vi "Signal Math (V1.00).vi"(0 "Time Data":refnum<class "GSwFormDSP.lvclass">, 5 "error in (no error)":errorcluster, 7 "Application Name":string="SigMath", 9 "State Queue":T2[](array[typedef])=["SC >>> Initialize"]) -> (19 "error out":errorcluster)   [LabVIEW 2022 SP3, in "SigMath.lvclass"]
uses:
  SigMath.lvclass
  API/Generic Utilities_class/utils/GenUtil State List.ctl
  API/GSwFormDSP_class/GSwFormDSP.lvclass
  <vilib>/Utility/sysdir.llb/System Directory Type.ctl
  W:/projects/archives/23 Charette AI Group/SPWB/API/Generic Utilities_class/Generic Utilities.lvclass
  <vilib>/Platform/browser.llb/Open URL in Default Browser (path).vi
  <vilib>/addons/_AddQ/G#Object/G#Object.lvclass
  API/Generic Utilities_class/Generic Utilities.lvclass
panel:
  in  "Operation":T1(tab)
  in  "Add Signals":bool
  in  "Add - Select Signals":i32[](listbox) caption="Select Signals"
  in  "Deconvolute Signals":bool
  in  "Convolute Signals":bool
  in  "Substract Signals":bool
  in  "Sub Signals A":i32[](listbox) caption="Select Signals (Set A)"
  in  "Sub Signals B":i32[](listbox) caption="Select Signals (Set B)"
  out "Measured Delay (Samples)":dbl
  out "Measured Delay (msec)":dbl
  in  "Weighting":u16(ring) items=["biased (N)", "unbiased (N-k)"]
  out "Cross Correlation Graph":cluster{"Ramp Pattern":dbl[], "Rxy":dbl[]}(graph)
  in  "X-Corr Signals A":i32[](listbox) caption="Select Signals (Set A)"
  in  "X-Corr Signals B":i32[](listbox) caption="Select Signals (Set B)"
  in  "AppData Folder":bool
  out "State History":string[](array[string])
  out "State Index":i32
  in  "Exit":bool
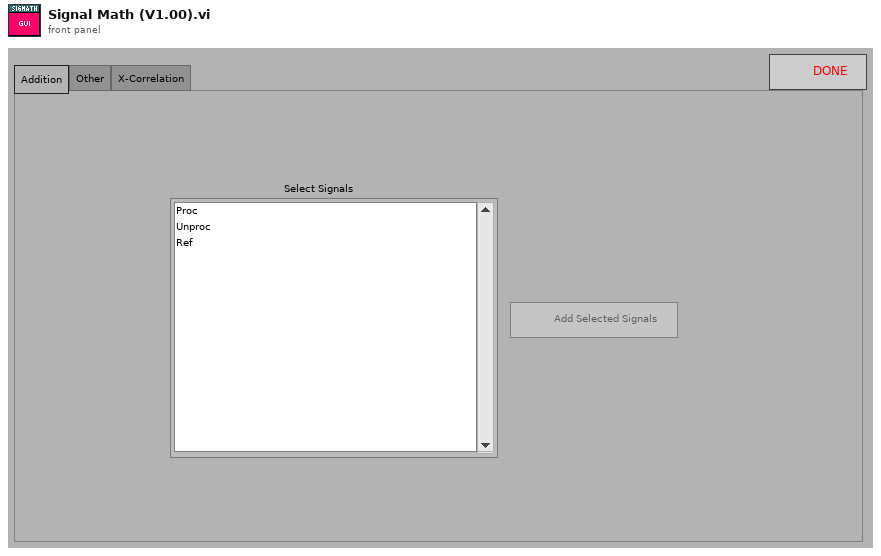
[diagram p1: front panel]
types:
  T1 = enum32{"Addition", "Other", "X-Correlation", "Settings"}
  T2 = typedef "Generic Utilities.lvclass/GenUtil State List.ctl" = string
  T3 = enum8{"Enabled", "Disabled", "Disabled and Grayed Out"}
  T4 = enum32{"Invalid", "Standard", "Closed", "Hidden", "Minimized", "Maximized"}
  T5 = typedef "System Directory Type.ctl" = i32
  T6 = typedef "SigMath.lvclass/SigMath Data.ctl" = cluster{"New Time Data Obj?":bool, "GSwFormDSP":refnum<class "GSwFormDSP.lvclass">}
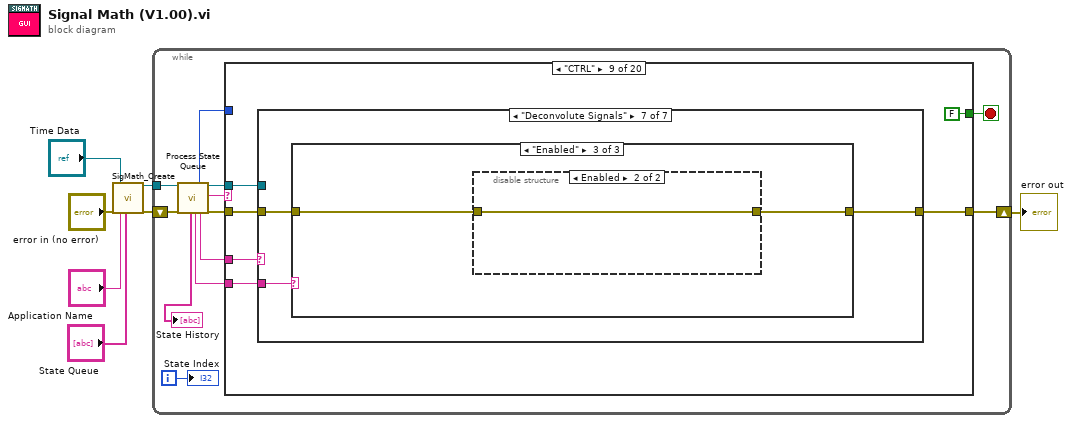
[diagram p0: block diagram]
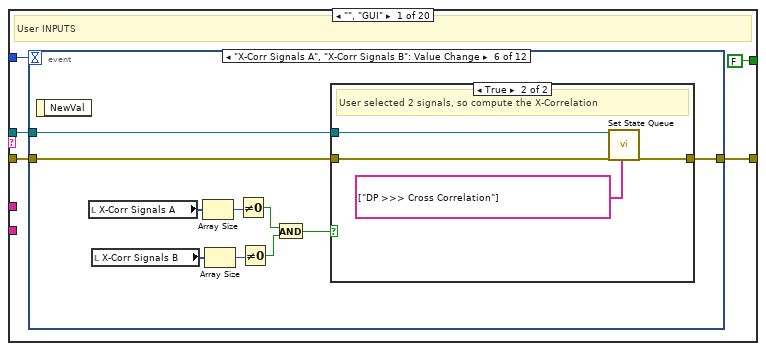
[diagram p2: hidden frame]
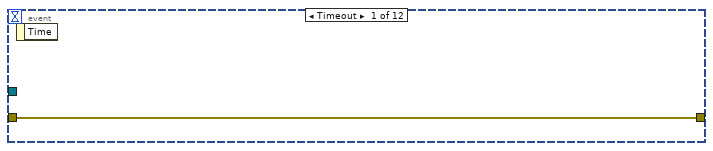
[diagram p3: hidden frame]
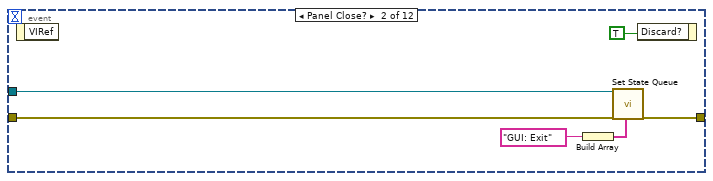
[diagram p4: hidden frame]
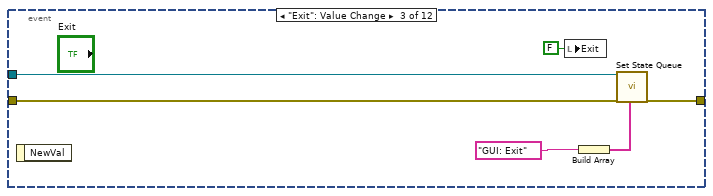
[diagram p5: hidden frame]
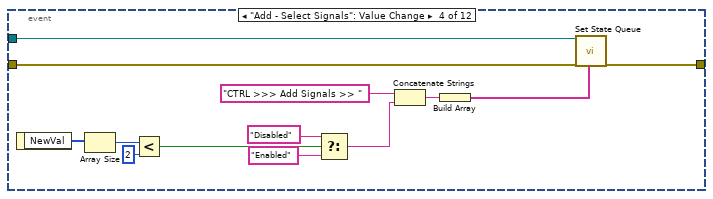
[diagram p6: hidden frame]
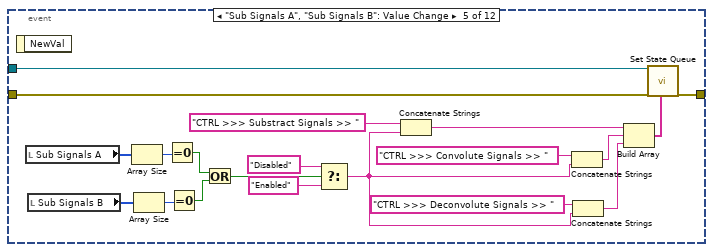
[diagram p7: hidden frame]
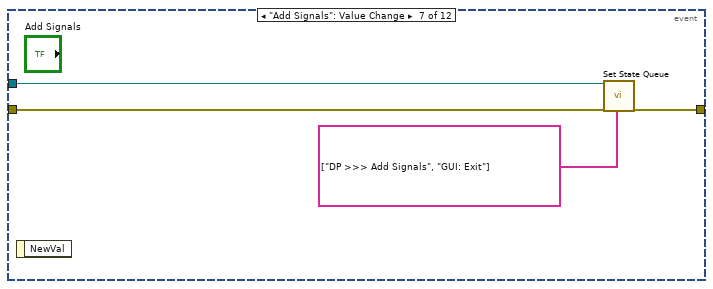
[diagram p9: hidden frame]
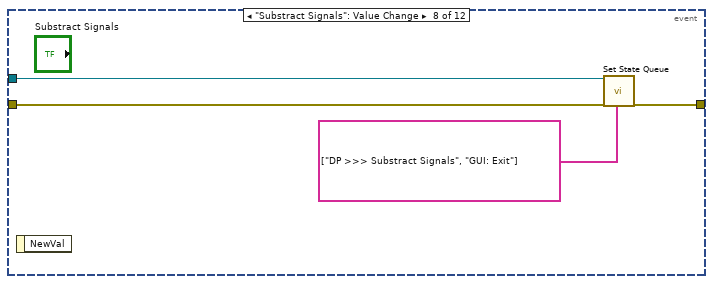
[diagram p10: hidden frame]
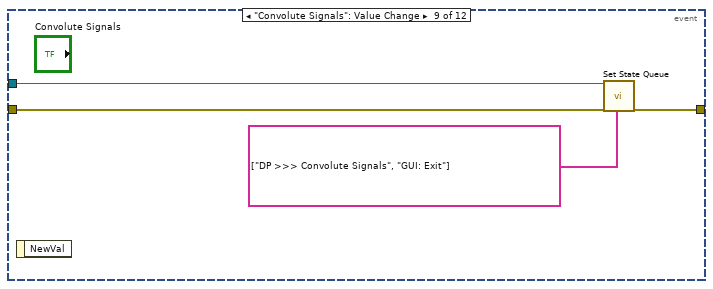
[diagram p11: hidden frame]
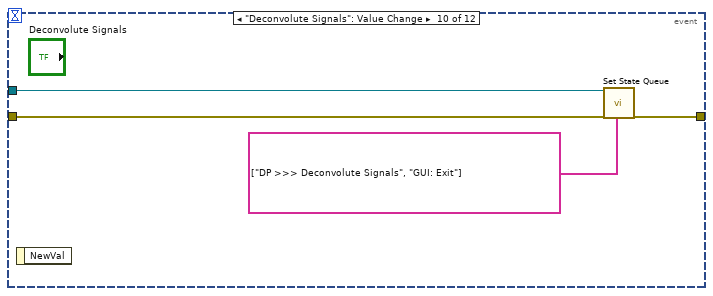
[diagram p12: hidden frame]
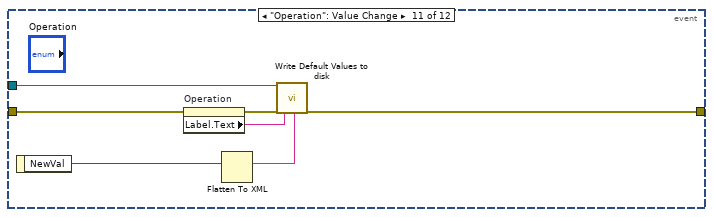
[diagram p13: hidden frame]
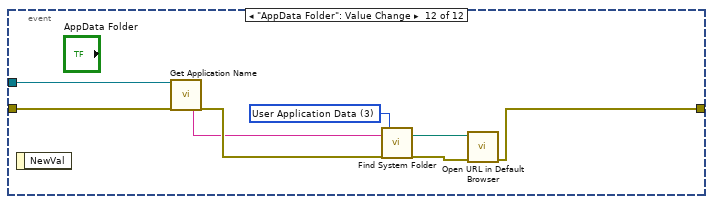
[diagram p14: hidden frame]
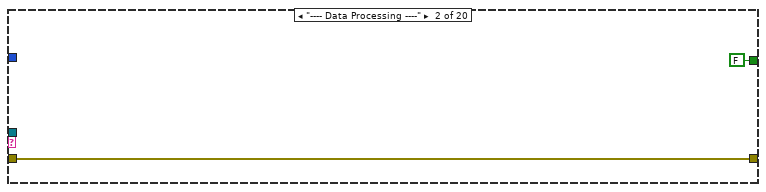
[diagram p15: hidden frame]
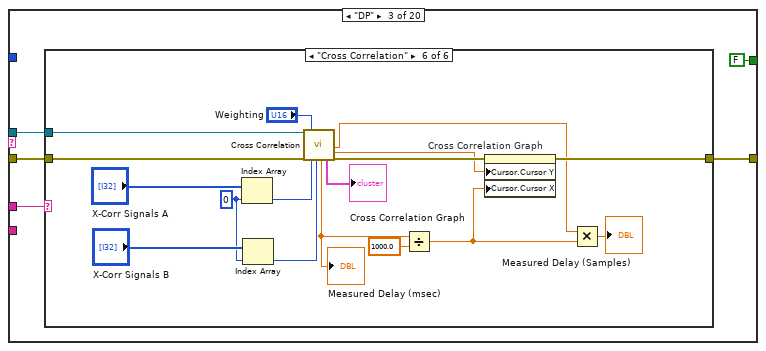
[diagram p16: hidden frame]
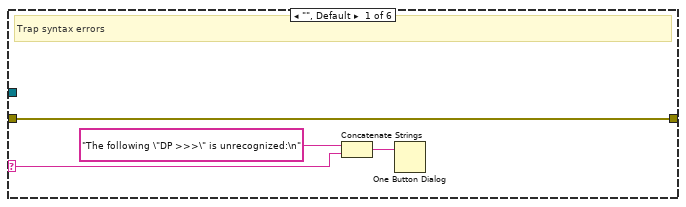
[diagram p17: hidden frame]
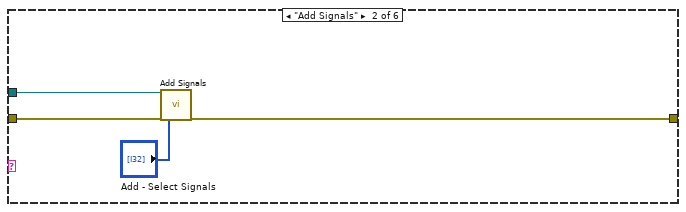
[diagram p18: hidden frame]
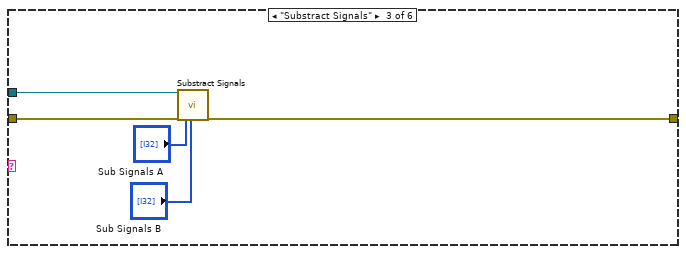
[diagram p19: hidden frame]
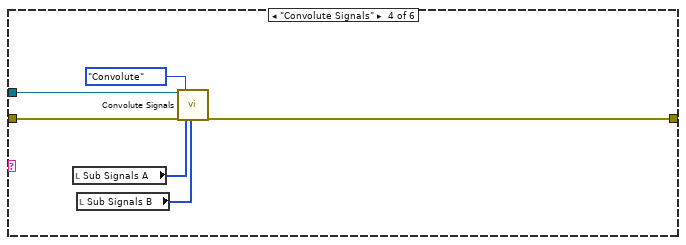
[diagram p20: hidden frame]
diagram:
  n1 = call "SigMath_Create.vi"("error in (no error)"="error in (no error)", "Time Data"="Time Data", "Application Name"="Application Name", "State Queue"="State Queue") -> ("reference out"=w7:refnum<class "SigMath.lvclass">, "error out"=w6:errorcluster)  [unwired: 14 in]
  n2 = while {
    shift-right: [w11] -> w2
    shift-left: w6 -> [w16]
    tunnel: w7 -> [w17]
    i -> [w18]
    stop <- w19 stop-if-true
    n3 = call "Process State Queue.vi"("reference in"=w17, "error in (no error)"=w16) -> ("State History"=→"State History":string[], "Additional Options"=w8:string, "Timeout"=w15:i32, "State Option"=w10:string, "reference out"=w14:refnum<class "SigMath.lvclass">, "Current State"=w13:string, "error out"=w12:errorcluster)  [unwired: 10 in, 1 out]
    n4 = case shown="\"CTRL\"" w13 {
      selector: w13 -> [_ _ _ _ _ _ _ _ _ _ _ _ _ _ _ _ w449 _ _ _]
      tunnel: w14 -> [w22 _ w119 _ w168 _ w184 _ w196 w317 _ w353 w372 w408 w433 _ _ _ _ w459]
      tunnel: [FALSE FALSE FALSE FALSE FALSE FALSE FALSE FALSE FALSE FALSE FALSE FALSE TRUE FALSE FALSE FALSE FALSE FALSE FALSE TRUE] -> w19
      tunnel: w15 -> [w23 _ _ _ _ _ _ _ _ _ _ _ _ _ _ _ _ _ _ _]
      tunnel: w10 -> [_ _ w122 _ w171 _ w180 _ w197 w314 _ _ _ w417 _ _ _ _ _ _]
      tunnel: w12 -> [w21 w117 w121 w166 w169 w177 w183 w191 w194 w316 w337 w350 w369 w407 w434 w445 w447 w452 w455 w458]
      tunnel: [w20 w117 w120 w166 w170 w177 w182 w191 w195 w315 w337 w342 w368 w405 w430 w445 w447 errorcluster {"status"=FALSE, "code"=0, "source"=""} ("error out") w455 w457] -> w11
      tunnel: w8 -> [_ _ _ _ _ _ _ _ w193 _ _ _ _ _ _ _ _ _ _ _]
      frame "", "GUI" {
        # "User INPUTS"
        n5 = event shown="[5] \"X-Corr Signals A\", \"X-Corr Signals B\": Value Change" {
          selector: _ -> [_ _ _ _ _ _ _ _ _ _ _ _]
          dyn-events: _ -> [_ _ _ _ _ _ _ _ _ _ _ _]
          timeout: w23 -> [_ _ _ _ _ _ _ _ _ _ _ _]
          tunnel: w22 -> [_ w30 w36 w47 w70 w80 w89 w93 w97 w101 w107 w115]
          tunnel: w21 -> [w25 w29 w34 w46 w69 w79 w88 w92 w96 w100 w104 w114]
          tunnel: [w25 w28 w35 w45 w68 w78 w87 w91 w95 w99 w102 w109] -> w20
          event Timeout {
            n6 = event-data() -> ()  [unwired: 1 in, 1 out]
          }
          event Panel Close? {
            n7 = event-data() -> ()  [unwired: 1 in, 1 out]
            n8 = Build Array(T2 "GUI: Exit" ("State List")) -> (w27:T2[])
            n9 = call "Set State Queue.vi"("reference in"=w30, "error in (no error)"=w29, "State Queue"=w27) -> ("error out"=w28:errorcluster)  [unwired: 15 in, 1 out]
            n10 = event-data("Discard?"=TRUE) -> ()  [unwired: 1 in, 1 out]
          }
          event "Exit": Value Change {
            n11 = event-data() -> ()  [unwired: 1 in, 1 out]
            n12 = local write "Exit"(FALSE ("Exit")) -> ()
            n13 = Build Array(T2 "GUI: Exit" ("State List")) -> (w33:T2[])
            n14 = call "Set State Queue.vi"("reference in"=w36, "error in (no error)"=w34, "State Queue"=w33) -> ("error out"=w35:errorcluster)  [unwired: 15 in, 1 out]
          }
          event "Add - Select Signals": Value Change {
            n15 = event-data() -> ("NewVal"=w50:i32[])  [unwired: 1 in]
            n16 = Array Size(array=w50) -> (size(s)=w49:i32)
            n17 = Less?(x=w49, y=2) -> (x < y?=w43:bool)
            n18 = Select(t="Disabled", s=w43, f="Enabled") -> (s? t:f=w40:string)
            n19 = Concatenate Strings("CTRL >>> Add Signals >> ", w40) -> (w39:string)
            n20 = Build Array(w39) -> (w38:string[])
            n21 = call "Set State Queue.vi"("reference in"=w47, "error in (no error)"=w46, "State Queue"=w38) -> ("error out"=w45:errorcluster)  [unwired: 15 in, 1 out]
          }
          event "Sub Signals A", "Sub Signals B": Value Change {
            n22 = event-data() -> ()  [unwired: 1 in, 1 out]
            n23 = local read "Sub Signals A"() -> (w61:i32[])
            n24 = local read "Sub Signals B"() -> (w60:i32[])
            n25 = Array Size(array=w61) -> (size(s)=w62:i32)
            n26 = Array Size(array=w60) -> (size(s)=w59:i32)
            n27 = Equal To 0?(x=w62) -> (x = 0?=w58:bool)
            n28 = Equal To 0?(x=w59) -> (x = 0?=w57:bool)
            n29 = Or(x=w58, y=w57) -> (x .or. y?=w56:bool)
            n30 = Select(t="Disabled", s=w56, f="Enabled") -> (s? t:f=w52:string)
            n31 = Concatenate Strings("CTRL >>> Substract Signals >> ", w52) -> (w64:string)
            n32 = Concatenate Strings("CTRL >>> Convolute Signals >> ", w52) -> (w54:string)
            n33 = Concatenate Strings("CTRL >>> Deconvolute Signals >> ", w52) -> (w51:string)
            n34 = Build Array(w64, w54, w51) -> (w63:string[])
            n35 = call "Set State Queue.vi"("reference in"=w70, "error in (no error)"=w69, "State Queue"=w63) -> ("error out"=w68:errorcluster)  [unwired: 15 in, 1 out]
          }
          event "X-Corr Signals A", "X-Corr Signals B": Value Change {
            n36 = event-data() -> ()  [unwired: 1 in, 1 out]
            n37 = local read "X-Corr Signals A"() -> (w76:i32[])
            n38 = local read "X-Corr Signals B"() -> (w75:i32[])
            n39 = Array Size(array=w76) -> (size(s)=w77:i32)
            n40 = Array Size(array=w75) -> (size(s)=w74:i32)
            n41 = Not Equal To 0?(x=w77) -> (x != 0?=w73:bool)
            n42 = Not Equal To 0?(x=w74) -> (x != 0?=w72:bool)
            n43 = And(x=w73, y=w72) -> (x .and. y?=w71:bool)
            n44 = case shown="True" w71 {
              tunnel: w80 -> [_ w85]
              tunnel: w79 -> [w81 w84]
              tunnel: [w81 w83] -> w78
              frame False {
                # "Less than 2 signals selected"
              }
              frame True {
                # "User selected 2 signals, so compute the X-Correlation"
                n45 = call "Set State Queue.vi"("reference in"=w85, "error in (no error)"=w84, "State Queue"=string[] ["DP >>> Cross Correlation"]) -> ("error out"=w83:errorcluster)  [unwired: 15 in, 1 out]
              }
            }
          }
          event "Add Signals": Value Change {
            n46 = event-data() -> ()  [unwired: 1 in, 1 out]
            n47 = call "Set State Queue.vi"("reference in"=w89, "error in (no error)"=w88, "State Queue"=string[] ["DP >>> Add Signals", "GUI: Exit"]) -> ("error out"=w87:errorcluster)  [unwired: 15 in, 1 out]
          }
          event "Substract Signals": Value Change {
            n48 = event-data() -> ()  [unwired: 1 in, 1 out]
            n49 = call "Set State Queue.vi"("reference in"=w93, "error in (no error)"=w92, "State Queue"=string[] ["DP >>> Substract Signals", "GUI: Exit"]) -> ("error out"=w91:errorcluster)  [unwired: 15 in, 1 out]
          }
          event "Convolute Signals": Value Change {
            n50 = event-data() -> ()  [unwired: 1 in, 1 out]
            n51 = call "Set State Queue.vi"("reference in"=w97, "error in (no error)"=w96, "State Queue"=string[] ["DP >>> Convolute Signals", "GUI: Exit"]) -> ("error out"=w95:errorcluster)  [unwired: 15 in, 1 out]
          }
          event "Deconvolute Signals": Value Change {
            n52 = event-data() -> ()  [unwired: 1 in, 1 out]
            n53 = call "Set State Queue.vi"("reference in"=w101, "error in (no error)"=w100, "State Queue"=string[] ["DP >>> Deconvolute Signals", "GUI: Exit"]) -> ("error out"=w99:errorcluster)  [unwired: 15 in, 1 out]
          }
          event "Operation": Value Change {
            n54 = event-data() -> ("NewVal"=w108:T1)  [unwired: 1 in]
            n55 = property on="Operation" class="TabCtl (strict)"(error in=w104) -> (error out=w103:errorcluster, "Label.Text"=w106:string)  [unwired: 1 in, 1 out]
            n56 = Flatten To XML(6:w108) -> (2:w105:string)
            n57 = call-dynamic "Write Default Values to disk.vi"("reference in"=w107, "error in (no error)"=w103, "Control Label"=w106, "Value (XML String)"=w105) -> ("error out"=w102:errorcluster)  [unwired: 14 in, 1 out]
          }
          event "AppData Folder": Value Change {
            w116 = T5 3 items=["User Home"=0, "User Desktop"=1, "User Documents"=2, "User Application Data"=3, "User Preferences"=4, "User Temporary"=5, "Public Documents"=6, "Public Application Data"=7, "Public Preferences"=8, "Public Cache"=13, "System Core Libraries"=9, "System Installed Libraries"=10, "Application Files"=11, "Boot Volume Root"=12] ("system directory type")
            n58 = event-data() -> ()  [unwired: 1 in, 1 out]
            n59 = call "Get Application Name.vi"("reference in"=w115, "error in (no error)"=w114) -> ("Application Name"=w112:string, "error out"=w113:errorcluster)  [unwired: 15 in, 1 out]
            n60 = call "Find System Folder.vi"("Application Name"=w112, "error in (no error)"=w113, "system directory type"=w116) -> ("System Folder"=w111:path, "error out"=w110:errorcluster)  [unwired: 15 in]
            n61 = call-poly <vilib>:"Open URL in Default Browser.vi"("error in (no error)"=w110, "path"=w111) -> ("error out"=w109:errorcluster)  [unwired: 4 in, 1 out]
          }
        }
      }
      frame "---- Data Processing ----" {
      }
      frame "DP" {
        n62 = case shown="\"Cross Correlation\"" w122 {
          selector: w122 -> [w125 _ _ _ _ _]
          tunnel: [w124 w129 w132 w140 w146 w155] -> w120
          tunnel: w121 -> [w124 w130 w135 w141 w147 w164]
          tunnel: w119 -> [_ w131 w136 w142 w148 w165]
          frame "", Default {
            # "Trap syntax errors"
            n63 = Concatenate Strings("The following \"DP >>>\" is unrecognized:\n", w125) -> (w126:string)
            n64 = One Button Dialog(message=w126) -> ()  [unwired: 1 in, 1 out]
          }
          frame "Add Signals" {
            n65 = call "Add Signals.vi"("reference in"=w131, "error in (no error)"=w130, "Select Signals"="Add - Select Signals") -> ("error out"=w129:errorcluster)  [unwired: 15 in, 1 out]
          }
          frame "Substract Signals" {
            n66 = call "Substract Signals.vi"("reference in"=w136, "error in (no error)"=w135, "Sub Signals A"="Sub Signals A", "Sub Signals B"="Sub Signals B") -> ("error out"=w132:errorcluster)  [unwired: 14 in, 1 out]
          }
          frame "Convolute Signals" {
            n67 = local read "Sub Signals A"() -> (w139:i32[])
            n68 = local read "Sub Signals B"() -> (w138:i32[])
            n69 = call "Convolute Signals.vi"("reference in"=w142, "error in (no error)"=w141, "Operation Option"=enum16{"Convolute", "DE-Convolute"}."Convolute", "Sub Signals A"=w139, "Sub Signals B"=w138) -> ("error out"=w140:errorcluster)  [unwired: 13 in, 1 out]
          }
          frame "Deconvolute Signals" {
            n70 = local read "Sub Signals A"() -> (w145:i32[])
            n71 = local read "Sub Signals B"() -> (w144:i32[])
            n72 = call "Convolute Signals.vi"("reference in"=w148, "error in (no error)"=w147, "Operation Option"=enum16{"Convolute", "DE-Convolute"}."DE-Convolute", "Sub Signals A"=w145, "Sub Signals B"=w144) -> ("error out"=w146:errorcluster)  [unwired: 13 in, 1 out]
          }
          frame "Cross Correlation" {
            w159 = 0 ("index")
            n73 = Index Array(array="X-Corr Signals A", index=w159) -> (element=w162:i32)
            n74 = Index Array(array="X-Corr Signals B", index=w159) -> (element=w160:i32)
            n75 = call "Cross Correlation.vi"("reference in"=w165, "error in (no error)"=w164, "Weighting"="Weighting", "Sub Signals A"=w162, "Sub Signals B"=w160) -> ("Delay (msec)"=w153:dbl, "correlogram"=→"Cross Correlation Graph":cluster{"Ramp Pattern":dbl[], "Rxy":dbl[]}, "Fs"=w150:dbl, "Max Amp"=w154:dbl, "error out"=w156:errorcluster)  [unwired: 9 in, 1 out]
            "Measured Delay (msec)" <- w153
            n76 = Divide(x=w153, y=1000.0) -> (x/y=w151:dbl)
            n77 = property on="Cross Correlation Graph" class="XYGraph (strict)"(error in=w156, "Cursor.Cursor Y"=w154, "Cursor.Cursor X"=w151) -> (error out=w155:errorcluster)  [unwired: 1 in, 1 out]
            n78 = Multiply(x=w150, y=w151) -> (x*y=→"Measured Delay (Samples)":dbl)
          }
        }
      }
      frame "---- Command ----" {
      }
      frame "CMD" {
        n79 = case shown="\"\", Default" w171 {
          selector: w171 -> [w174]
          tunnel: [w173] -> w170
          tunnel: w169 -> [w173]
          tunnel: w168 -> [_]
          frame "", Default {
            # "Trap syntax errors"
            n80 = Concatenate Strings("The following \"CMD >>>\" is unrecognized:\n", w174) -> (w175:string)
            n81 = One Button Dialog(message=w175) -> ()  [unwired: 1 in, 1 out]
          }
        }
      }
      frame "---- Scripts ----" {
      }
      frame "SC" {
        # "MUST ADD A COMMAND TO GUARANTEE THAT ALL THE SIGNALS HAVE THE SAME Fs???"
        n82 = case shown="\"Initialize\"" w180 {
          selector: w180 -> [w187 _]
          tunnel: [string[] [] ("State Queue OUT") string[] ["GUI: Initialize Ref", "CTRL >>> Task Tab", "CTRL >>> Signal List", "CTRL >>> Add Signals >> Disabled", "CTRL >>> Substract Signals >> Disabled", "CTRL >>> Convolute Signals >> Disabled", "CTRL >>> Deconvolute Signals >> Disabled", "FP >>> Open"] ("State Queue OUT")] -> w181
          frame "", Default {
            n83 = Concatenate Strings("The following \"Script\" is unrecognized:\n", w187) -> (w188:string)
            n84 = One Button Dialog(message=w188) -> ()  [unwired: 1 in, 1 out]
          }
          frame "Initialize" {
          }
        }
        n85 = call "Set State Queue.vi"("reference in"=w184, "error in (no error)"=w183, "State Queue Options"=enum16{"Replace", "Append", "Prepend"}."Prepend", "State Queue"=w181) -> ("error out"=w182:errorcluster)  [unwired: 14 in, 1 out]
      }
      frame "---- Front Panel Mgmt ----" {
      }
      frame "CTRL" {
        n86 = case shown="\"Deconvolute Signals\"" w197 {
          selector: w197 -> [w201 _ _ _ _ _ _]
          tunnel: w196 -> [_ w209 w230 _ _ _ _]
          tunnel: [w199 w204 w223 w257 w270 w283 w299] -> w195
          tunnel: w194 -> [w199 w207 w229 w256 w269 w282 w298]
          tunnel: w193 -> [_ _ _ w258 w271 w284 w300]
          frame "unknown", Default {
            n87 = Concatenate Strings("The following control name is unrecognized:\n", w201) -> (w200:string)
            n88 = One Button Dialog(message=w200) -> ()  [unwired: 1 in, 1 out]
          }
          frame "Task Tab" {
            n89 = property on="Operation" class="TabCtl (strict)"(error in=w207) -> (error out=w208:errorcluster, "Label.Text"=w206:string, "Value"=w211:T1)  [unwired: 1 in, 1 out]
            n90 = call-dynamic "Read Default Values from Disk.vi"("reference in"=w209, "error in (no error)"=w208, "Control Label"=w206) -> ("Value (XML String)"=w203:string, "error out"=w205:errorcluster)  [unwired: 14 in, 1 out]
            n91 = case shown="\"\"" w203 {
              selector: w203 -> [w218 _]
              tunnel: [w213 w220] -> w212
              tunnel: w211 -> [w215 w220]
              tunnel: w205 -> [w216 w219]
              tunnel: [w216 w219] -> w210
              frame "anything", Default {
                n92 = Unflatten From XML(xml string=w218, type=w215, error in (no error)=w216) -> (value=w214:T1, error out=w217:errorcluster)
                n93 = Select(t=w215, s=w217, f=w214) -> (s? t:f=w213:T1)
              }
              frame "" {
                # "Either the file was not found or there was some error"
              }
            }
            n94 = property on="Operation" class="TabCtl (strict)"(error in=w210, "Value"=w212) -> (error out=w204:errorcluster)  [unwired: 1 in, 1 out]
          }
          frame "Signal List" {
            n95 = call "Get - SigMath Data.vi"("reference in"=w230, "error in (no error)"=w229) -> ("SigMath Data"=w228:T6, "error out"=w226:errorcluster)  [unwired: 15 in, 1 out]
            n96 = Unbundle By Name(w228) -> ("GSwFormDSP"=w227:refnum<class "GSwFormDSP.lvclass">)
            n97 = call-dynamic "Get - Names and Units.vi"("reference in"=w227, "error in (no error)"=w226) -> ("Signal Names"=w225:string[], "error out"=w224:errorcluster)  [unwired: 13 in, 3 out]
            n98 = for {
              N: 5 -> [_]
              tunnel: w225 -> [w235]
              tunnel: i32[] [] ("Select Signals") -> [w232]
              shift-right: [w233] -> w223
              shift-left: w224 -> [w234]
              i -> [w231]
              n99 = case shown="4" w231 {
                tunnel: w235 -> [w239 w243 w247 w251 w255]
                tunnel: w234 -> [w238 w242 w246 w250 w254]
                tunnel: [w237 w241 w245 w249 w253] -> w233
                tunnel: w232 -> [w236 w240 w244 w248 w252]
                frame 0, Default {
                  n100 = property on="Add - Select Signals" class="LstBox (strict)"(error in=w238, "Item Names"=w239, "Value"=w236) -> (error out=w237:errorcluster)  [unwired: 1 in, 1 out]
                }
                frame 1 {
                  n101 = property on="Sub Signals A" class="LstBox (strict)"(error in=w242, "Item Names"=w243, "Value"=w240) -> (error out=w241:errorcluster)  [unwired: 1 in, 1 out]
                }
                frame 2 {
                  n102 = property on="Sub Signals B" class="LstBox (strict)"(error in=w246, "Item Names"=w247, "Value"=w244) -> (error out=w245:errorcluster)  [unwired: 1 in, 1 out]
                }
                frame 3 {
                  n103 = property on="X-Corr Signals A" class="LstBox (strict)"(error in=w250, "Item Names"=w251, "Value"=w248) -> (error out=w249:errorcluster)  [unwired: 1 in, 1 out]
                }
                frame 4 {
                  n104 = property on="X-Corr Signals B" class="LstBox (strict)"(error in=w254, "Item Names"=w255, "Value"=w252) -> (error out=w253:errorcluster)  [unwired: 1 in, 1 out]
                }
              }
            }
          }
          frame "Add Signals" {
            n105 = case shown="\"\", Default" w258 {
              selector: w258 -> [w260 _ _]
              tunnel: [w259 w264 w267] -> w257
              tunnel: w256 -> [w259 w265 w268]
              frame "", Default {
                n106 = Concatenate Strings("The following \"Add Signals\" control option is unrecognized:\n", w260) -> (w261:string)
                n107 = One Button Dialog(message=w261) -> ()  [unwired: 1 in, 1 out]
              }
              frame "Disabled" {
                n108 = property on="Add Signals" class="Bool"(error in=w265, "DisabledEnum"=T3."Disabled and Grayed Out" ("Disabled")) -> (error out=w264:errorcluster)  [unwired: 1 in, 1 out]
              }
              frame "Enabled" {
                n109 = property on="Add Signals" class="Bool"(error in=w268, "DisabledEnum"=T3."Enabled" ("Disabled")) -> (error out=w267:errorcluster)  [unwired: 1 in, 1 out]
              }
            }
          }
          frame "Substract Signals" {
            n110 = case shown="\"\", Default" w271 {
              selector: w271 -> [w273 _ _]
              tunnel: [w272 w277 w280] -> w270
              tunnel: w269 -> [w272 w278 w281]
              frame "", Default {
                n111 = Concatenate Strings("The following \"Substract Signals\" control option is unrecognized:\n", w273) -> (w274:string)
                n112 = One Button Dialog(message=w274) -> ()  [unwired: 1 in, 1 out]
              }
              frame "Disabled" {
                n113 = property on="Substract Signals" class="Bool"(error in=w278, "DisabledEnum"=T3."Disabled and Grayed Out" ("Disabled")) -> (error out=w277:errorcluster)  [unwired: 1 in, 1 out]
              }
              frame "Enabled" {
                n114 = property on="Substract Signals" class="Bool"(error in=w281, "DisabledEnum"=T3."Enabled" ("Disabled")) -> (error out=w280:errorcluster)  [unwired: 1 in, 1 out]
              }
            }
          }
          frame "Convolute Signals" {
            n115 = case shown="\"Enabled\"" w284 {
              selector: w284 -> [w286 _ _]
              tunnel: [w285 w290 w292] -> w283
              tunnel: w282 -> [w285 w291 w293]
              frame "", Default {
                n116 = Concatenate Strings("The following \"Convolute Signals\" control option is unrecognized:\n", w286) -> (w287:string)
                n117 = One Button Dialog(message=w287) -> ()  [unwired: 1 in, 1 out]
              }
              frame "Disabled" {
                n118 = property on="Convolute Signals" class="Bool"(error in=w291, "DisabledEnum"=T3."Disabled and Grayed Out" ("Disabled")) -> (error out=w290:errorcluster)  [unwired: 1 in, 1 out]
              }
              frame "Enabled" {
                n119 = disable-structure shown="Enabled" {
                  disable-tunnel: w293 -> [w296 w297]
                  disable-tunnel: [w295 w297] -> w292
                  frame Disabled {
                    n120 = property on="Convolute Signals" class="Bool"(error in=w296, "DisabledEnum"=T3."Enabled" ("Disabled")) -> (error out=w295:errorcluster)  [unwired: 1 in, 1 out]
                  }
                  frame Enabled {
                  }
                }
              }
            }
          }
          frame "Deconvolute Signals" {
            n121 = case shown="\"Enabled\"" w300 {
              selector: w300 -> [w302 _ _]
              tunnel: [w301 w306 w308] -> w299
              tunnel: w298 -> [w301 w307 w309]
              frame "", Default {
                n122 = Concatenate Strings("The following \"Deconvolute Signals\" control option is unrecognized:\n", w302) -> (w303:string)
                n123 = One Button Dialog(message=w303) -> ()  [unwired: 1 in, 1 out]
              }
              frame "Disabled" {
                n124 = property on="Deconvolute Signals" class="Bool"(error in=w307, "DisabledEnum"=T3."Disabled and Grayed Out" ("Disabled")) -> (error out=w306:errorcluster)  [unwired: 1 in, 1 out]
              }
              frame "Enabled" {
                n125 = disable-structure shown="Enabled" {
                  disable-tunnel: w309 -> [w312 w313]
                  disable-tunnel: [w311 w313] -> w308
                  frame Disabled {
                    n126 = property on="Deconvolute Signals" class="Bool"(error in=w312, "DisabledEnum"=T3."Enabled" ("Disabled")) -> (error out=w311:errorcluster)  [unwired: 1 in, 1 out]
                  }
                  frame Enabled {
                  }
                }
              }
            }
          }
        }
      }
      frame "FP" {
        n127 = case shown="\"Open\"" w314 {
          selector: w314 -> [w319 _]
          tunnel: w317 -> [_ w327]
          tunnel: w316 -> [w320 w326]
          tunnel: [w320 w323] -> w315
          frame "unknown", Default {
            n128 = Concatenate Strings("The following FP Command name is unrecognized:\n", w319) -> (w321:string)
            n129 = One Button Dialog(message=w321) -> ()  [unwired: 1 in, 1 out]
          }
          frame "Open" {
            n130 = call-dynamic "Get VI Ref.vi"("reference in"=w327, "error in (no error)"=w326) -> ("GUI VI Ref"=w324:refnum<vi>, "error out"=w325:errorcluster)  [unwired: 14 in, 2 out]
            n131 = property class="VI"(reference=w324, error in=w325) -> (reference out=w329:refnum<vi>, error out=w330:errorcluster, "Front Panel.Open"=w328:bool)
            n132 = case shown="False" w328 {
              tunnel: [w333 w336] -> w323
              tunnel: w330 -> [w332 w336]
              tunnel: w329 -> [w331 _]
              frame False {
                n133 = invoke class="VI" method="FP.Open"(reference=w331, error in=w332, "Activate"=TRUE, "State"=T4."Standard") -> (error out=w333:errorcluster)  [unwired: 1 in, 4 out]
              }
              frame True {
              }
            }
          }
        }
      }
      frame "---- GUI Functions ----" {
      }
      frame "GUI: Initialize Ref" {
        n134 = control-ref of="GUI Reference"() -> (w349:refnum<vi>)
        n135 = disable-structure shown="Disabled" {
          frame Enabled {
          }
          frame Disabled {
            w355 = string[] [] ("Item Names")
            n136 = property on="Add - Select Signals" class="LstBox (strict)"("Item Names"=w355) -> ()  [unwired: 2 in, 2 out]
            n137 = property on="Sub Signals A" class="LstBox (strict)"("Item Names"=w355) -> ()  [unwired: 2 in, 2 out]
            n138 = property on="Sub Signals B" class="LstBox (strict)"("Item Names"=w355) -> ()  [unwired: 2 in, 2 out]
          }
        }
        n139 = call "Set VI Ref.vi"("reference in"=w353, "error in (no error)"=w350, "ReInit All to Default?"=FALSE, "GUI VI Ref"=w349) -> ("reference out"=w352:refnum<class "SigMath.lvclass">, "error out"=w348:errorcluster)  [unwired: 14 in]
        n140 = call "Set Close Panel (Yes or No).vi"("reference in"=w352, "error in (no error)"=w348) -> ("reference out"=w351:refnum<class "SigMath.lvclass">, "error out"=w347:errorcluster)  [unwired: 16 in]
        n141 = call "Set Message Window Ref.vi"("reference in"=w351, "error in (no error)"=w347) -> ("reference out"=w346:refnum<class "SigMath.lvclass">, "error out"=w345:errorcluster)  [unwired: 16 in]
        n142 = call "Get - SigMath Data.vi"("reference in"=w346, "error in (no error)"=w345) -> ("SigMath Data"=w344:T6, "error out"=w341:errorcluster)  [unwired: 15 in, 1 out]
        n143 = Unbundle By Name(w344) -> ("GSwFormDSP"=w340:refnum<class "GSwFormDSP.lvclass">, "New Time Data Obj?"=w343:bool)
        n144 = case shown="True" w343 {
          tunnel: [w356 w359] -> w342
          tunnel: w341 -> [w356 w357]
          tunnel: w340 -> [_ w358]
          frame False {
          }
          frame True {
            n145 = call "Set - wForms.vi"("reference in"=w358, "error in (no error)"=w357, "Init wForms"=TRUE) -> ("error out"=w359:errorcluster)  [unwired: 15 in, 1 out]
          }
        }
      }
      frame "GUI: Exit" {
        n146 = call-dynamic "Get Message Window Ref.vi"("reference in"=w372, "error in (no error)"=w369) -> ("reference out"=w371:refnum<class "SigMath.lvclass">, "Msg Win Ref"=w367:refnum<vi>, "error out"=w370:errorcluster)  [unwired: 15 in]
        n147 = call-dynamic "Get VI Ref.vi"("reference in"=w371, "error in (no error)"=w370) -> ("reference out"=w375:refnum<class "SigMath.lvclass">, "GUI VI Ref"=w373:refnum<vi>, "error out"=w374:errorcluster)  [unwired: 14 in, 1 out]
        n148 = call-dynamic "Get Close Panel (Yes or No).vi"("reference in"=w375, "error in (no error)"=w374) -> ("Close Panel?"=w376:bool, "reference out"=w365:refnum<class "SigMath.lvclass">, "error out"=w366:errorcluster)  [unwired: 15 in]
        n149 = call-dynamic "Get OBJ NOT RefNum.vi"("reference in"=w365, "error in (no error)"=w366) -> ("OBJ not a refnum?"=w364:bool, "reference out"=w363:refnum<class "SigMath.lvclass">, "error out"=w362:errorcluster)  [unwired: 15 in]
        n150 = case shown="True" w364 {
          tunnel: [w381 w384] -> w361
          tunnel: w363 -> [_ w383]
          tunnel: w362 -> [w381 w382]
          frame False {
            # "The OBJ already exist, indicating this is a dialog box or sub-vi so do NOT destroy the original OBJ."
          }
          frame True {
            # "New OBJ was created, so it needs to be deleted."
            n151 = call-dynamic "Destroy.vi"("reference in"=w383, "error in (no error)"=w382) -> ("error out"=w385:errorcluster)  [unwired: 16 in, 1 out]
            n152 = disable-structure shown="Disabled" {
              disable-tunnel: w385 -> [w387 w388]
              disable-tunnel: [w386 w388] -> w384
              frame Disabled {
                # "Enable when NEEDED"
                n153 = call <vilib>:"GarbageCollector.vi"("error in (no error)"=w387) -> ("error out"=w386:errorcluster)  [unwired: 16 in, 2 out]
              }
              frame Enabled {
              }
            }
          }
        }
        n154 = Close Reference(reference=w367, error in (no error)=w361) -> (error out=w379:errorcluster)
        n155 = case shown="True" w376 {
          tunnel: w379 -> [w390 w394]
          tunnel: [w390 w393] -> w377
          tunnel: [w389 w392] -> w378
          tunnel: w373 -> [w389 w391]
          frame False {
          }
          frame True {
            n156 = property class="VI"(reference=w391, error in=w394) -> (reference out=w396:refnum<vi>, error out=w395:errorcluster, "Front Panel.Open"=w397:bool)
            n157 = case shown="True" w397 {
              tunnel: [w399 w403] -> w393
              tunnel: w395 -> [w399 w402]
              tunnel: w396 -> [w398 w401]
              tunnel: [w398 w400] -> w392
              frame False {
              }
              frame True {
                n158 = invoke class="VI" method="FP.Close"(reference=w401, error in=w402) -> (reference out=w400:refnum<vi>, error out=w403:errorcluster)  [unwired: 1 in, 1 out]
              }
            }
          }
        }
        n159 = Close Reference(reference=w378, error in (no error)=w377) -> (error out=w368:errorcluster)
      }
      frame "SEND MSG" {
        n160 = call-dynamic "Get Message Window Ref.vi"("reference in"=w408, "error in (no error)"=w407) -> ("Msg Win Ref"=w404:refnum<vi>, "error out"=w406:errorcluster)  [unwired: 15 in, 1 out]
        n161 = property class="VI"(reference=w404, error in=w406) -> (reference out=w410:refnum<vi>, error out=w409:errorcluster, "Front Panel.Open"=w411:bool)
        n162 = case shown="False" w411 {
          tunnel: [w425 w429] -> w413
          tunnel: w409 -> [w420 w429]
          tunnel: w410 -> [w422 w428]
          tunnel: [w424 w428] -> w412
          frame False {
            w423 = FALSE ("Wait Until Done")
            n163 = invoke class="VI" method="Run VI"(reference=w422, error in=w420, "Wait until done"=w423, "Auto Dispose Ref"=w423) -> (reference out=w421:refnum<vi>, error out=w419:errorcluster)  [unwired: 1 in, 3 out]
            n164 = invoke class="VI" method="FP.Open"(reference=w421, error in=w419, "Activate"=TRUE, "State"=T4."Standard") -> (reference out=w424:refnum<vi>, error out=w425:errorcluster)  [unwired: 1 in, 3 out]
          }
          frame True {
          }
        }
        n165 = Concatenate Strings("\r\n", w417) -> (w416:string)
        n166 = invoke class="VI" method="Ctrl Val.Set"(reference=w412, error in=w413, "Control Name"="Message", "Value"=w416) -> (error out=w405:errorcluster)  [unwired: 1 in, 4 out]
      }
      frame "CLOSE MSG" {
        n167 = call-dynamic "Get Message Window Ref.vi"("reference in"=w433, "error in (no error)"=w434) -> ("Msg Win Ref"=w431:refnum<vi>, "error out"=w432:errorcluster)  [unwired: 15 in, 1 out]
        n168 = property class="VI"(reference=w431, error in=w432) -> (reference out=w436:refnum<vi>, error out=w437:errorcluster, "Front Panel.Open"=w435:bool)
        n169 = case shown="True" w435 {
          tunnel: [w439 w440] -> w430
          tunnel: w437 -> [w439 w444]
          tunnel: w436 -> [_ w443]
          frame False {
          }
          frame True {
            n170 = invoke class="VI" method="FP.Close"(reference=w443, error in=w444) -> (reference out=w442:refnum<vi>, error out=w441:errorcluster)  [unwired: 1 in, 1 out]
            n171 = invoke class="VI" method="Abort VI"(reference=w442, error in=w441) -> (error out=w440:errorcluster)  [unwired: 1 in, 2 out]
          }
        }
      }
      frame "---- Miscelleneous ----" {
      }
      frame "unknown", Default {
        n172 = Concatenate Strings("The following state is unrecognized?\n", w449) -> (w448:string)
        n173 = One Button Dialog(message=w448) -> ()  [unwired: 1 in, 1 out]
      }
      frame "Error" {
        n174 = call <vilib>:"General Error Handler.vi"("error in (no error)"=w452) -> ()  [unwired: 10 in, 5 out]
      }
      frame "Next" {
        # "This is an empty case used so the queue does NOT stop if there is an empty string between two valid states!"
      }
      frame "Quit" {
        # "WARNING!, If the state machine crash, then it will also \"Quit\"??"
        # "This is the case used to simply exit when this GUI is used as a SubVI!"
        n175 = call-dynamic "Destroy.vi"("reference in"=w459, "error in (no error)"=w458) -> ("error out"=w457:errorcluster)  [unwired: 16 in, 1 out]
      }
    }
    "State Index" <- w18
  }
  "error out" <- w2
